vi "Set Vecto Config Version.vi"(8 "error in (no error)":errorcluster, 10 "Cfg Version":string, 11 "VolatusAPI in":refnum<class "VolatusAPI.lvclass">) -> (0 "error out":errorcluster, 3 "VolatusAPI out":refnum<class "VolatusAPI.lvclass">)   [LabVIEW 2020, in "Volatus.lvlib" / "VolatusAPI.lvclass"]
uses:
  VolatusAPI.lvclass
  VolatusAPI.lvclass/VolatusAPI.ctl
  lv-vecto/Vecto/Vecto/Vecto.lvclass
  lv-vecto/Vecto/DiscoveryService/DiscoveryService.lvclass
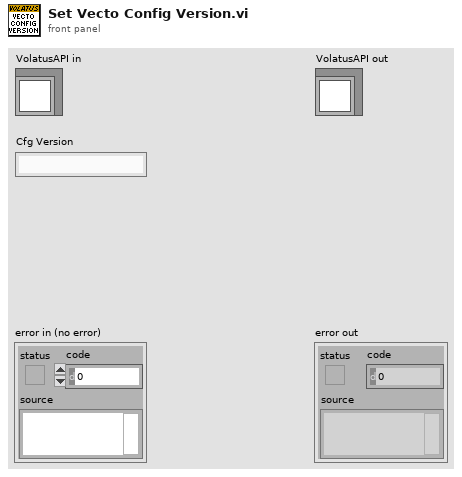
[diagram p1: front panel]
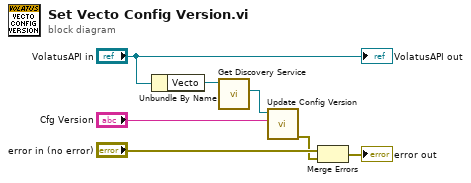
[diagram p0: block diagram]
diagram:
  n1 = Unbundle By Name("VolatusAPI in") -> ("Vecto"=w5:refnum<class "Vecto.lvclass">)
  n2 = call "Get Discovery Service.vi"("Vecto in"=w5) -> ("DiscoveryService"=w4:refnum<class "DiscoveryService.lvclass">)  [unwired: 8 in, 2 out]
  n3 = call "Update Config Version.vi"("Cfg Version"="Cfg Version", "NodeDiscovery in"=w4) -> ("error out"=w1:errorcluster)  [unwired: 8 in, 1 out]
  n4 = Merge Errors("error in (no error)", w1) -> (→"error out":errorcluster)
  "VolatusAPI out" <- "VolatusAPI in"
